vi "lock-in data transfer 0.3 copy.vi"(4 "points in buffer":i32=256, 5 "string":string="\n", 6 "number of points":dbl=617.0) -> (1 "Average\n[Y.0]":dbl, 2 "Average\n[X, R]":dbl, 3 "Array x":dbl[](array[numeric])=[0.0002212534, 0.0002746601, 0.0002899189, 0.0002365122, 0.0002441425, 0.0002555866, 0.0002059946, 0.0002021799, 0.0002594013, 0.0002594013, 0.0002288828, 0.0002708454, 0.0002937336, 0.0002479572, 0.0002365122, 0.000263216, 0.0002174387, 0.0001792917, 0.0002212534, 0.0002594013, 0.0002326975, 0.0002441425, 0.0002899189, 0.0002708454, 0.0002365122, 0.0002441425, 0.0002746601, 0.0002365122, 0.0002250681, 0.0002746601, 0.0002746601, 0.0002403269, 0.0002746601, 0.0002861042, 0.0002365122, 0.000213624, 0.0002555866, 0.0002250681, 0.0002174387, 0.0002937336, 0.000263216, 0.0002212534, 0.0002670307, 0.0003166217, 0.0002288828, 0.0002212534, 0.0002746601, 0.0003242511, 0.0002174387, 0.0002288828, 0.0003318805, 0.0002899189, 0.0002059946, 0.0002822895, 0.0002899189, 0.000213624, 0.0002098093, 0.000263216, 0.0002365122, 0.0002212534, 0.0002899189, 0.0002937336, 0.0002479572, 0.0002403269, 0.0002937336, 0.0002670307, 0.0002059946, 0.0002365122, 0.0002861042, 0.0002517719, 0.0002403269, 0.0002975482, 0.0002784748, 0.0002326975, 0.000263216, 0.0002861042, 0.000213624, 0.0001869211, 0.0002365122, 0.0002288828, 0.0002021799, 0.000263216, 0.0002861042, 0.0002365122, 0.0002403269, 0.0002937336, 0.0002708454, 0.0002326975, 0.000263216, 0.0002594013, 0.0002250681, 0.0002365122, 0.0002975482, 0.0002555866, 0.0002250681, 0.0002517719, 0.0002403269, 0.0002021799, 0.0002174387, 0.0002403269, 0.0002288828, 0.000213624, 0.000263216, 0.0002899189, 0.0002479572, 0.0002479572, 0.000263216, 0.0002365122, 0.0001831064, 0.0002441425, 0.0002746601, 0.0002365122, 0.0002441425, 0.0002975482, 0.0002670307, 0.0002212534, 0.0002403269, 0.0002517719, 0.0002098093, 0.0001945505, 0.0002288828, 0.0002326975, 0.0002326975, 0.0002784748, 0.0002861042, 0.0002403269, 0.0002479572, 0.0002822895, 0.0002517719, 0.0002098093, 0.0002670307, 0.0002784748, 0.0002365122, 0.0002517719, 0.0002975482, 0.0002746601, 0.0002365122, 0.0002555866, 0.0001983652, 0.000213624, 0.0002326975, 0.0002594013, 0.0002899189, 0.0002403269, 0.0002517719, 0.0003051776, 0.0002441425, 0.000263216, 0.0002746601, 0.0002555866, 0.0002326975, 0.0002365122, 0.000263216, 0.0002670307, 0.0002670307, 0.0002517719, 0.0002670307, 0.0002365122, 0.0002479572, 0.0002670307, 0.0002365122, 0.0002098093, 0.0002670307, 0.0002937336, 0.0002365122, 0.0002670307, 0.0002937336, 0.0002059946, 0.0002365122, 0.000312807, 0.0002403269, 0.0002174387, 0.0002784748, 0.0002899189, 0.0002250681, 0.0002746601, 0.000312807, 0.0002708454, 0.0002098093, 0.0002822895, 0.0003013629, 0.0002098093, 0.0002288828, 0.0003051776, 0.000263216, 0.0002288828, 0.0002822895, 0.0002822895, 0.0002365122, 0.0002365122, 0.0002937336, 0.0002594013, 0.0002288828, 0.0002899189, 0.0002937336, 0.0002365122, 0.0002479572, 0.0002861042, 0.0002365122, 0.000213624, 0.000263216, 0.0002670307, 0.0002288828, 0.000263216, 0.0002937336, 0.0002594013, 0.0002441425, 0.0002822895, 0.000263216, 0.0002021799, 0.000213624, 0.0002517719, 0.0002365122, 0.0002212534, 0.0002708454, 0.0002937336, 0.0002441425, 0.0002555866, 0.0002861042, 0.0002365122, 0.0002250681, 0.0002441425, 0.0002555866, 0.000213624, 0.0002517719, 0.0002861042, 0.0002555866, 0.0002365122, 0.0002670307, 0.0002479572, 0.0002059946, 0.0002479572, 0.0002746601, 0.0002326975, 0.0002250681, 0.0002899189, 0.0002746601, 0.0002441425, 0.000263216, 0.0002784748, 0.000213624, 0.0002098093, 0.0002555866, 0.000263216, 0.0002288828, 0.000263216, 0.0002784748, 0.0002441425, 0.0002288828, 0.0002708454, 0.000263216, 0.0001831064, 0.000213624, 0.0002441425, 0.0002594013, 0.0002555866, 0.0002670307, 0.0002708454, 0.0001869211, 0.000263216, 0.0003166217, 0.0002288828, 0.000213624, 0.0002975482, 0.0002822895, 0.0002212534, 0.0002861042, 0.0003089923, 0.0002326975, 0.0001945505, 0.0002250681, 0.0002975482, 0.0002212534, 0.0002250681, 0.0002708454, 0.0002784748, 0.0002365122, 0.000263216, 0.000312807, 0.0002365122, 0.0002365122, 0.0002899189, 0.0002670307, 0.000213624, 0.0002937336, 0.0002899189, 0.000213624, 0.0002441425, 0.0002899189, 0.0002403269, 0.0002250681, 0.0003013629, 0.0002899189, 0.0002250681, 0.0002365122, 0.0002899189, 0.000263216, 0.0002441425, 0.0002746601, 0.0002746601, 0.0002403269, 0.0002517719, 0.0002861042, 0.0002746601, 0.0002174387, 0.0003051776, 0.000312807, 0.0002365122, 0.0002403269, 0.0003013629, 0.0002670307, 0.0001983652, 0.0002861042, 0.0002784748, 0.0001945505, 0.0002517719, 0.0003089923, 0.0002326975, 0.0002288828, 0.000312807, 0.0003013629, 0.0002098093, 0.000263216, 0.0002784748, 0.0002517719, 0.000213624, 0.0002479572, 0.0003013629, 0.0002479572, 0.000213624, 0.0002746601, 0.0002365122, 0.0002059946, 0.0002365122, 0.0002670307, 0.0002288828, 0.0002174387, 0.0002822895, 0.000263216, 0.0002365122, 0.0002899189, 0.0002555866, 0.0002021799, 0.0002288828, 0.0002670307, 0.0002212534, 0.0002250681, 0.0002822895, 0.0002746601, 0.0002098093, 0.000263216, 0.0002746601, 0.0002098093, 0.0001907358, 0.0002441425, 0.0002479572, 0.0001945505, 0.0002555866, 0.0003051776, 0.0002365122, 0.0002365122, 0.0002784748, 0.0002479572, 0.0002098093, 0.0002403269, 0.0002746601, 0.0002326975, 0.0002441425, 0.0003013629, 0.0002784748, 0.0002212534, 0.0002517719, 0.0002594013, 0.0002059946, 0.0001983652, 0.0002555866, 0.0002594013, 0.0002365122, 0.000263216, 0.0002937336, 0.000263216, 0.0002479572, 0.0002784748, 0.0002555866, 0.0002288828, 0.0002479572, 0.0002708454, 0.0002365122, 0.0002555866, 0.0002746601, 0.0002555866, 0.0002288828, 0.0002517719, 0.0002670307, 0.0002212534, 0.0002326975, 0.0002594013, 0.0002555866, 0.0002326975, 0.0002746601, 0.0002899189, 0.0002517719, 0.0002288828, 0.0002670307, 0.0002403269, 0.0002174387, 0.000263216, 0.0002899189, 0.0002403269, 0.0002555866, 0.0002899189, 0.0002670307, 0.0002250681, 0.0002822895, 0.0002021799, 0.0001640329, 0.0002899189, 0.0002708454, 0.0001831064, 0.0002670307, 0.0003089923, 0.0002555866, 0.0002288828, 0.0002784748, 0.0002670307, 0.0002365122, 0.0002326975, 0.0002517719, 0.0002479572, 0.0002594013, 0.0002441425, 0.0002708454, 0.000263216, 0.0001831064, 0.0002517719, 0.0003242511, 0.0002059946, 0.0002479572, 0.0002746601, 0.0002365122, 0.0002555866, 0.0002937336, 0.0002708454, 0.0002250681, 0.0002555866, 0.0002746601, 0.0002098093, 0.0002365122, 0.0002937336, 0.0002594013, 0.000213624, 0.0002670307, 0.0002784748, 0.0002059946, 0.0002098093, 0.0003013629, 0.0002326975, 0.0001487741, 0.0002746601, 0.0002937336, 0.0002174387, 0.0002441425, 0.0002708454, 0.0002365122, 0.0002212534, 0.0002021799, 0.0001831064, 0.0002746601, 0.0002746601, 0.0002098093, 0.0002708454, 0.0002822895, 0.0002403269, 0.0002365122, 0.0002250681, 0.0001602182, 0.0002517719, 0.0002098093, 0.0002174387, 0.0002098093, 0.0002670307, 0.0002937336, 0.0002174387, 0.0002746601, 0.0002975482, 0.0002326975, 0.0002212534, 0.0002594013, 0.0002479572, 0.0002174387, 0.0002670307, 0.0002861042, 0.0002326975, 0.0002441425, 0.0002784748, 0.0002441425, 0.0002212534, 0.0002555866, 0.0002594013, 0.0002365122, 0.0002479572, 0.0002899189, 0.0002555866, 0.0002365122, 0.0002670307, 0.0002708454, 0.0002326975, 0.0002479572, 0.0002899189, 0.0002517719, 0.0002326975, 0.0002822895, 0.0002899189, 0.0002365122, 0.0002517719, 0.0002822895, 0.0002594013, 0.000213624, 0.0002746601, 0.0002861042, 0.0002365122, 0.0002594013, 0.0002937336, 0.0002555866, 0.0002250681, 0.0002822895, 0.0002861042, 0.0002250681, 0.0002517719, 0.0002975482, 0.0002555866, 0.0002365122, 0.0002899189, 0.000263216, 0.0002250681, 0.0002517719, 0.0002365122, 0.0002174387, 0.000263216, 0.0002746601, 0.0002708454, 0.0002326975, 0.0002479572, 0.0002822895, 0.0002708454, 0.0002250681, 0.0002365122, 0.0002594013, 0.0002365122, 0.0002479572, 0.0002517719, 0.0002784748, 0.000263216, 0.0002212534, 0.0002365122, 0.0002326975, 0.000263216, 0.0002594013, 0.0001869211, 0.0001831064, 0.0002899189, 0.0002899189, 0.000213624, 0.0002670307, 0.0002937336, 0.0001716623, 0.0001716623, 0.0003051776, 0.0002708454, 0.0001831064, 0.0002517719, 0.0002937336, 0.0002365122, 0.0002365122, 0.000263216, 0.0001792917, 0.0002098093, 0.0002212534, 0.000213624, 0.0002403269, 0.0001907358, 0.0002517719, 0.0002822895, 0.0002479572, 0.0002365122, 0.000263216, 0.0002288828, 0.0002365122, 0.000263216, 0.0002517719, 0.0002403269, 0.0002517719, 0.0002708454, 0.0002555866, 0.0001907358, 0.0002861042, 0.0002365122, 0.0001029973, 0.0002555866, 0.0003471393, 0.0001869211, 0.0002212534, 0.0003318805, 0.0002822895, 0.0002059946, 0.0002937336, 0.0003051776, 0.0001945505, 0.0002059946, 0.0003166217, 0.0002822895, 0.0001907358, 0.0002899189, 0.0002899189, 0.0001831064, 0.0002365122, 0.0002899189] format="%#_9e")   [LabVIEW 2010]
uses:
  Instance           1 38Saved   lock-in data transfer 0.3 copy .vi
  Instance           3 38Saved   lock-in data transfer 0.3 copy .vi
  Instance           2 38Saved   lock-in data transfer 0.3 copy .vi
  Instance           7 38Saved   lock-in data transfer 0.3 copy .vi
  Instance           6 38Saved   lock-in data transfer 0.3 copy .vi
  Instance          10 38Saved   lock-in data transfer 0.3 copy .vi
  Instance           5 38Saved   lock-in data transfer 0.3 copy .vi
  Instance           4 38Saved   lock-in data transfer 0.3 copy .vi
panel:
  out "Array y":dbl[](array[numeric])
  out "read \nbuffer 2":string="2.899189e-004,2.365122e-004,2.517719e-004,2.822895e-004,2.594013e-004,2.136240e-004,2.746601e-004,2.861042e-004,2.365122e-004,2.594013e-004,2.937336e-004,2.555866e-004,2.250681e-004,2.822895e-004,2.861042e-004,2.250681e-004,2.517719e-004,2.975482e-004,2.555866e-004,2.365122e-004,2.899189e-004,2.632160e-004,2.250681e-004,2.517719e-004,2.365122e-004,2.174387e-004,2.632160e-004,2.746601e-004,2.708454e-004,2.326975e-004,2.479572e-004,2.822895e-004,2.708454e-004,2.250681e-004,2.365122e-004,2.594013e-004,2.365122e-004,2.479572e-004,2.517719e-004,2.784748e-004,2.632160e-004,2.212534e-004,2.365122e-004,2.326975e-004,2.632160e-004,2.594013e-004,1.869211e-004,1.831064e-004,2.899189e-004,2.899189e-004,2.136240e-004,2.670307e-004,2.937336e-004,1.716623e-004,1.716623e-004,3.051776e-004,2.708454e-004,1.831064e-004,2.517719e-004,2.937336e-004,2.365122e-004,2.365122e-004,2.632160e-004,1.792917e-004,2.098093e-004,2.212534e-004,2.136240e-004,2.403269e-004,1.907358e-004,2.517719e-004,2.822895e-004,2.479572e-004,2.365122e-004,2.632160e-004,2.288828e-004,2.365122e-004,2.632160e-004,2.517719e-004,2.403269e-004,2.517719e-004,2.708454e-004,2.555866e-004,1.907358e-004,2.861042e-004,2.365122e-004,1.029973e-004,2.555866e-004,3.471393e-004,1.869211e-004,2.212534e-004,3.318805e-004,2.822895e-004,2.059946e-004,2.937336e-004,3.051776e-004,1.945505e-004,2.059946e-004,3.166217e-004,2.822895e-004,1.907358e-004,2.899189e-004,2.899189e-004,1.831064e-004,2.365122e-004,2.899189e-004,\n"
  out "read\nbuffer":string="2.899189e-004,2.365122e-004,2.517719e-004,2.822895e-004,2.594013e-004,2.136240e-004,2.746601e-004,2.861042e-004,2.365122e-004,2.594013e-004,2.937336e-004,2.555866e-004,2.250681e-004,2.822895e-004,2.861042e-004,2.250681e-004,2.517719e-004,2.975482e-004,2.555866e-004,2.365122e-004,2.899189e-004,2.632160e-004,2.250681e-004,2.517719e-004,2.365122e-004,2.174387e-004,2.632160e-004,2.746601e-004,2.708454e-004,2.326975e-004,2.479572e-004,2.822895e-004,2.708454e-004,2.250681e-004,2.365122e-004,2.594013e-004,2.365122e-004,2.479572e-004,2.517719e-004,2.784748e-004,2.632160e-004,2.212534e-004,2.365122e-004,2.326975e-004,2.632160e-004,2.594013e-004,1.869211e-004,1.831064e-004,2.899189e-004,2.899189e-004,2.136240e-004,2.670307e-004,2.937336e-004,1.716623e-004,1.716623e-004,3.051776e-004,2.708454e-004,1.831064e-004,2.517719e-004,2.937336e-004,2.365122e-004,2.365122e-004,2.632160e-004,1.792917e-004,2.098093e-004,2.212534e-004,2.136240e-004,2.403269e-004,1.907358e-004,2.517719e-004,2.822895e-004,2.479572e-004,2.365122e-004,2.632160e-004,2.288828e-004,2.365122e-004,2.632160e-004,2.517719e-004,2.403269e-004,2.517719e-004,2.708454e-004,2.555866e-004,1.907358e-004,2.861042e-004,2.365122e-004,1.029973e-004,2.555866e-004,3.471393e-004,1.869211e-004,2.212534e-004,3.318805e-004,2.822895e-004,2.059946e-004,2.937336e-004,3.051776e-004,1.945505e-004,2.059946e-004,3.166217e-004,2.822895e-004,1.907358e-004,2.899189e-004,2.899189e-004,1.831064e-004,2.365122e-004,2.899189e-004,\n"
  out "size":i32=617
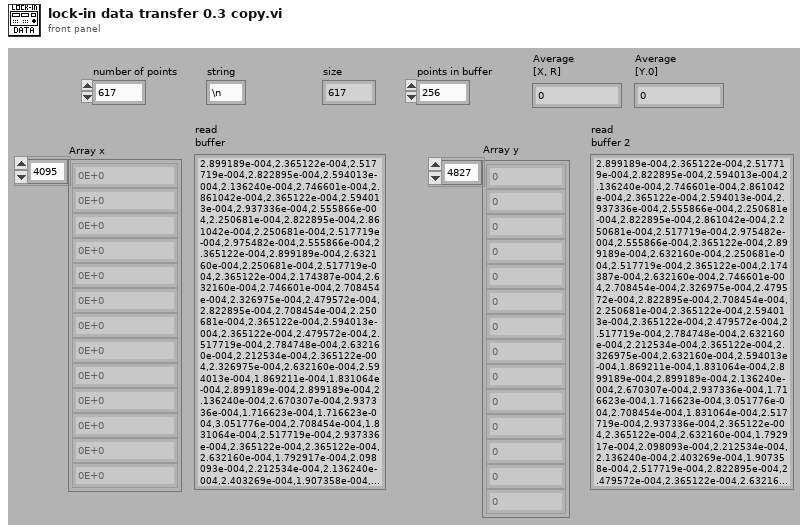
[diagram p1: front panel]
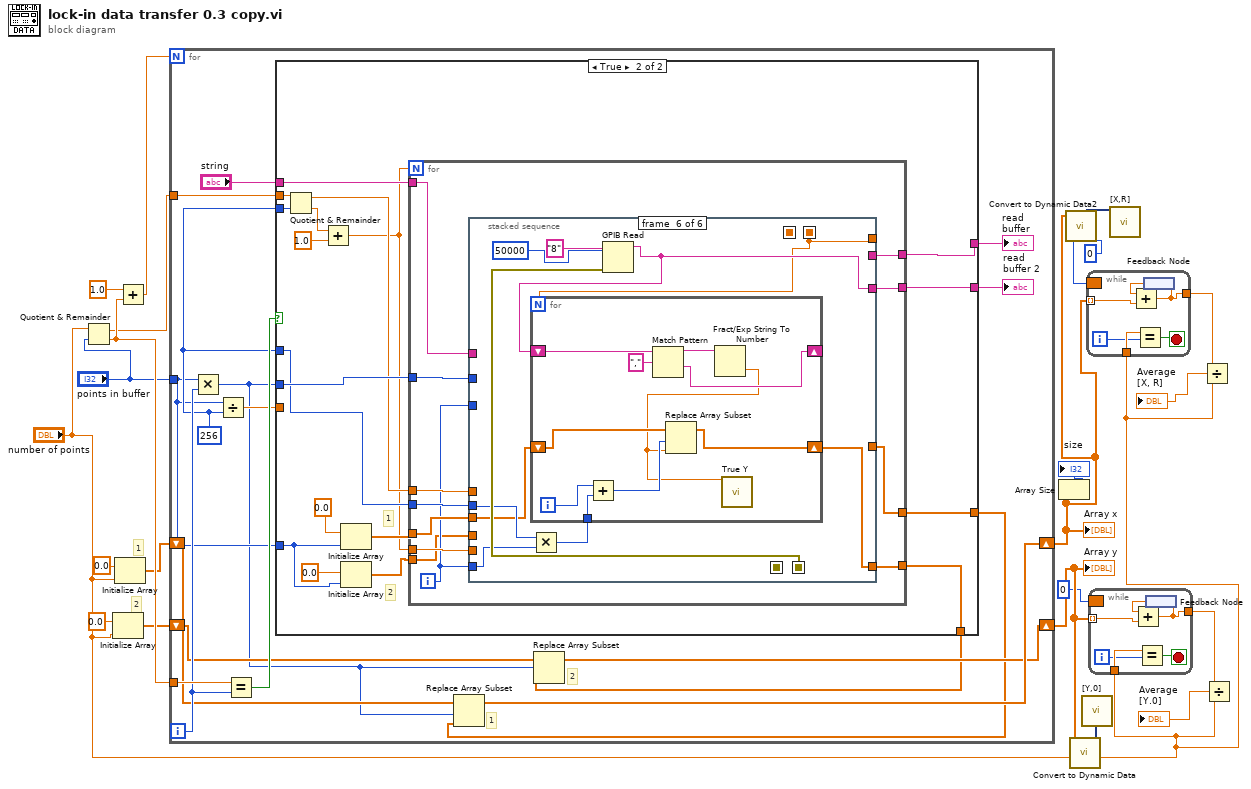
[diagram p0: block diagram]
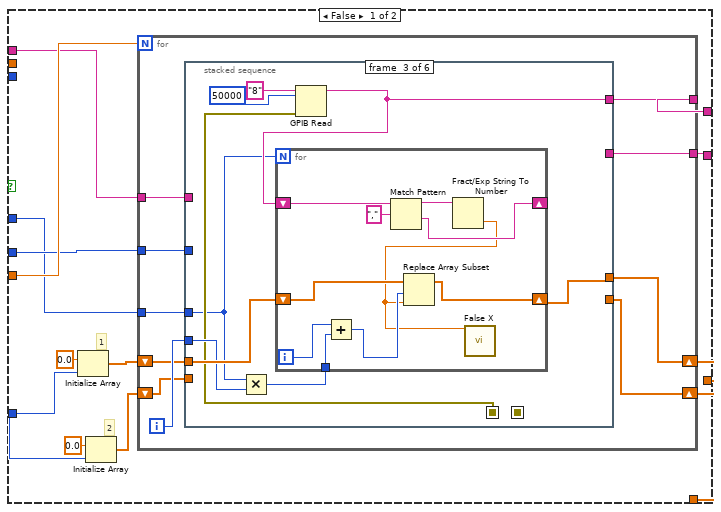
[diagram p2: hidden frame]
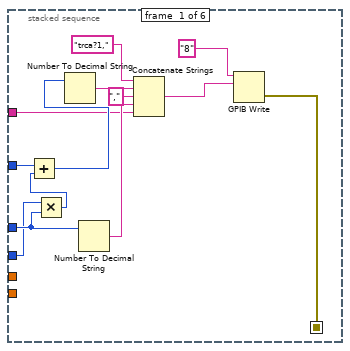
[diagram p3: hidden frame]
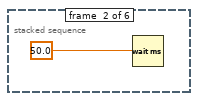
[diagram p4: hidden frame]
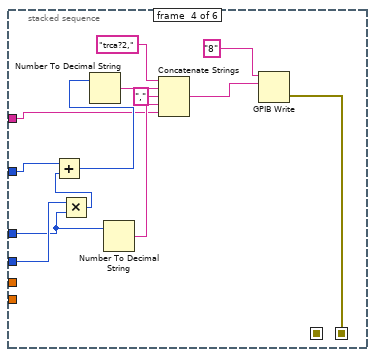
[diagram p5: hidden frame]
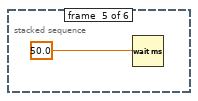
[diagram p6: hidden frame]
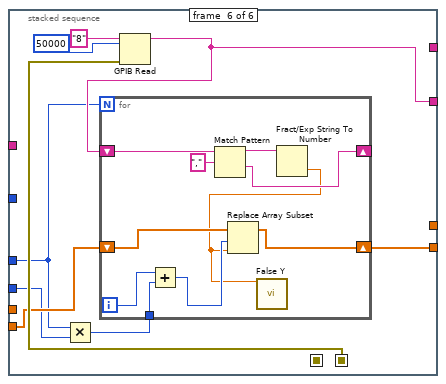
[diagram p7: hidden frame]
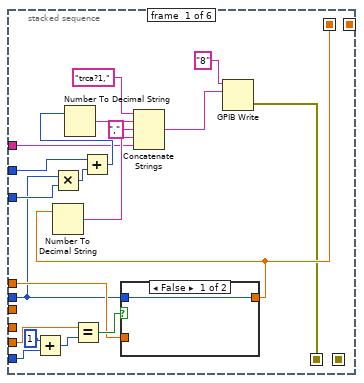
[diagram p8: hidden frame]
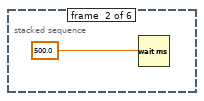
[diagram p10: hidden frame]
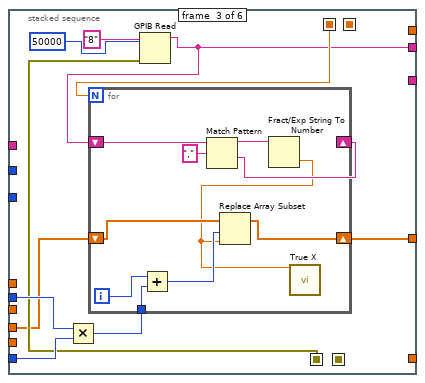
[diagram p11: hidden frame]
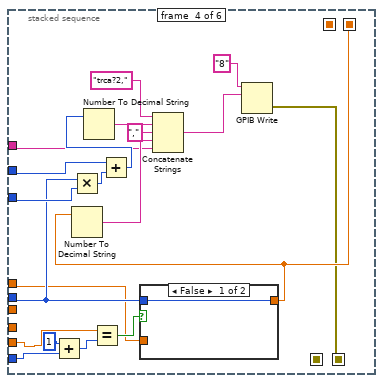
[diagram p12: hidden frame]
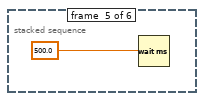
[diagram p14: hidden frame]
diagram:
  # "2"
  # "1"
  n1 = Quotient & Remainder(x="number of points", y="points in buffer") -> (x-y*floor(x/y)=w14:dbl, floor(x/y)=w19:dbl)
  n2 = Initialize Array(0.0 ("element"), "number of points") -> (w12:dbl[])
  n3 = Initialize Array(0.0 ("element"), "number of points") -> (w16:dbl[])
  n4 = Add(x=1.0, y=w19) -> (x+y=w20:dbl)
  n5 = for {
    N: w20 -> [_]
    tunnel: "points in buffer" -> [w30]
    tunnel: w19 -> [w38]
    shift-right: [w35] -> w7
    shift-left: w16 -> [w36]
    tunnel: w14 -> [w33]
    shift-right: [w26] -> w10
    shift-left: w12 -> [w27]
    i -> [w37]
    w32 = 256
    # "2"
    # "1"
    n6 = Multiply(x=w30, y=w37) -> (x*y=w25:i32)
    n7 = Divide(x=w30, y=w32) -> (x/y=w31:dbl)
    n8 = Equal?(x=w38, y=w37) -> (x = y?=w34:bool)
    n9 = case shown="True" w34 {
      tunnel: w32 -> [w48 w138]
      tunnel: w33 -> [_ w145]
      tunnel: w32 -> [_ w144]
      tunnel: w31 -> [w51 _]
      tunnel: w25 -> [w50 w143]
      tunnel: [w47 w136] -> w22
      tunnel: w30 -> [w41 w132]
      tunnel: "string" -> [w46 w135]
      tunnel: [w45 w134] -> w28
      tunnel: [w43 w128] -> w24
      tunnel: [w39 w130] -> w23
      frame False {
        # "2"
        # "1"
        n10 = Initialize Array(0.0 ("element"), w41) -> (w44:dbl[])
        n11 = Initialize Array(0.0 ("element"), w41) -> (w40:dbl[])
        n12 = for {
          N: w51 -> [_]
          tunnel: w48 -> [w60]
          tunnel: w50 -> [w59]
          tunnel: w46 -> [w58]
          tunnel: [w57] -> w45
          shift-right: [w53] -> w47
          shift-left: w44 -> [w56]
          tunnel: [w55] -> w43
          shift-right: [w52] -> w39
          shift-left: w40 -> [w54]
          i -> [w61]
          n13 = stacked-sequence {
            seq-local: [w62 _ _ _ _ _] -> [_ _ w79 _ _ _]
            seq-local: [_ _ _ w95 _ _] -> [_ _ _ _ _ w113]
            tunnel: w61 -> [w69 _ w82 w97 _ w110]
            tunnel: w56 -> [_ _ w84 _ _ _]
            tunnel: [_ _ w83 _ _ _] -> w53
            tunnel: w60 -> [w70 _ w76 w96 _ w111]
            tunnel: w59 -> [w68 _ _ w98 _ _]
            tunnel: w58 -> [w65 _ _ w99 _ _]
            tunnel: [_ _ w78 _ _ _] -> w57
            tunnel: [_ _ _ _ _ w114] -> w55
            tunnel: w54 -> [_ _ _ _ _ w112]
            tunnel: [_ _ _ _ _ w109] -> w52
            frame #0 {
              n14 = Multiply(x=w69, y=w70) -> (x*y=w67:i32)
              n15 = Add(x=w68, y=w67) -> (x+y=w66:i32)
              n16 = Number To Decimal String(number=w66) -> (decimal integer string=w73:string)  [unwired: 1 out]
              n17 = Number To Decimal String(number=w70) -> (decimal integer string=w71:string)  [unwired: 1 out]
              n18 = Concatenate Strings("trca?1,", w73, "," ("string"), w71, w65) -> (w63:string)
              n19 = GPIB Write(0:"8", 1:w63) -> (6:w62:errorcluster)  [unwired: 1 in, 3 out]
            }
            frame #1 {
              n20 = Wait (ms)(milliseconds to wait=50.0 ("x")) -> ()  [unwired: 1 out]
            }
            frame #2 {
              n21 = Multiply(x=w76, y=w82) -> (x*y=w81:i32)
              n22 = GPIB Read(0:"8", 1:50000, 3:w79) -> (5:w78:string)  [unwired: 4 out]
              n23 = for {
                N: w76 -> [_]
                shift-right: [w90] -> _
                shift-left: w78 -> [w92]
                shift-right: [w89] -> w83
                shift-left: w84 -> [w91]
                tunnel: w81 -> [w88]
                i -> [w87]
                n24 = Add(x=w87, y=w88) -> (x+y=w86:i32)
                n25 = Match Pattern(string=w92, regular expression=",") -> (before substring=w94:string, after substring=w90:string)  [unwired: 3 out]
                n26 = Fract/Exp String To Number(string=w94) -> (number=w85:dbl)  [unwired: 4 out]
                n27 = Replace Array Subset(array=w91, new element=w85, index=w86) -> (w89:dbl[])
                n28 = call "False X"("Signals"=w85) -> ()  [unwired: 6 in, 13 out]
              }
            }
            frame #3 {
              n29 = Multiply(x=w97, y=w96) -> (x*y=w104:i32)
              n30 = Add(x=w98, y=w104) -> (x+y=w105:i32)
              n31 = Number To Decimal String(number=w105) -> (decimal integer string=w101:string)  [unwired: 1 out]
              n32 = Number To Decimal String(number=w96) -> (decimal integer string=w103:string)  [unwired: 1 out]
              n33 = Concatenate Strings("trca?2,", w101, "," ("string"), w103, w99) -> (w107:string)
              n34 = GPIB Write(0:"8", 1:w107) -> (6:w95:errorcluster)  [unwired: 1 in, 3 out]
            }
            frame #4 {
              n35 = Wait (ms)(milliseconds to wait=50.0 ("x")) -> ()  [unwired: 1 out]
            }
            frame #5 {
              n36 = Multiply(x=w111, y=w110) -> (x*y=w117:i32)
              n37 = GPIB Read(0:"8", 1:50000, 3:w113) -> (5:w114:string)  [unwired: 4 out]
              n38 = for {
                N: w111 -> [_]
                shift-right: [w123] -> _
                shift-left: w114 -> [w125]
                shift-right: [w122] -> w109
                shift-left: w112 -> [w124]
                tunnel: w117 -> [w121]
                i -> [w120]
                n39 = Add(x=w120, y=w121) -> (x+y=w119:i32)
                n40 = Match Pattern(string=w125, regular expression=",") -> (before substring=w127:string, after substring=w123:string)  [unwired: 3 out]
                n41 = Fract/Exp String To Number(string=w127) -> (number=w118:dbl)  [unwired: 4 out]
                n42 = Replace Array Subset(array=w124, new element=w118, index=w119) -> (w122:dbl[])
                n43 = call "False Y"("Signals"=w118) -> ()  [unwired: 6 in, 13 out]
              }
            }
          }
        }
      }
      frame True {
        # "2"
        # "1"
        n44 = Quotient & Remainder(x=w145, y=w144) -> (x-y*floor(x/y)=w141:dbl, floor(x/y)=w140:dbl)
        n45 = Add(x=w140, y=1.0) -> (x+y=w129:dbl)
        n46 = Initialize Array(0.0 ("element"), w132) -> (w137:dbl[])
        n47 = Initialize Array(0.0 ("element"), w132) -> (w131:dbl[])
        n48 = for {
          N: w129 -> [_]
          tunnel: w143 -> [w157]
          tunnel: w129 -> [w155]
          tunnel: w138 -> [w154]
          tunnel: w141 -> [w153]
          tunnel: w137 -> [w156]
          tunnel: [w147] -> w136
          tunnel: w135 -> [w151]
          tunnel: [w150] -> w134
          tunnel: [w149] -> w128
          tunnel: w131 -> [w148]
          tunnel: [w146] -> w130
          i -> [w152]
          n49 = stacked-sequence {
            seq-local: [w158 _ _ _ _ _] -> [_ _ w186 _ _ _]
            seq-local: [w162 _ _ _ _ _] -> [_ _ w184 _ _ _]
            seq-local: [_ _ _ w203 _ _] -> [_ _ _ _ _ w225]
            seq-local: [_ _ _ w202 _ _] -> [_ _ _ _ _ w230]
            tunnel: w157 -> [w164 _ _ w208 _ _]
            tunnel: w156 -> [_ _ _ _ _ w224]
            tunnel: [_ _ w181 _ _ _] -> w147
            tunnel: w152 -> [w173 _ w189 w201 _ w226]
            tunnel: w155 -> [w170 _ _ w206 _ _]
            tunnel: w154 -> [w166 _ w190 w205 _ w229]
            tunnel: w153 -> [w168 _ _ w204 _ _]
            tunnel: w152 -> [w167 _ _ w207 _ _]
            tunnel: w151 -> [w161 _ _ w209 _ _]
            tunnel: [_ _ w182 _ _ _] -> w150
            tunnel: [_ _ _ _ _ w228] -> w149
            tunnel: w148 -> [_ _ w183 _ _ _]
            tunnel: [_ _ _ _ _ w227] -> w146
            tunnel: [_ _ _ _ _ w225] -> _
            frame #0 {
              n50 = Add(x=1, y=w173) -> (x+y=w171:i32)
              n51 = Multiply(x=w166, y=w167) -> (x*y=w165:i32)
              n52 = Equal?(x=w170, y=w171) -> (x = y?=w169:bool)
              n53 = Add(x=w164, y=w165) -> (x+y=w163:i32)
              n54 = Number To Decimal String(number=w163) -> (decimal integer string=w176:string)  [unwired: 1 out]
              n55 = case shown="False" w169 {
                tunnel: [w178 w179] -> w162
                tunnel: w166 -> [w178 _]
                tunnel: w168 -> [_ w179]
                frame False {
                }
                frame True {
                }
              }
              n56 = Number To Decimal String(number=w162) -> (decimal integer string=w174:string)  [unwired: 1 out]
              n57 = Concatenate Strings("trca?1,", w176, "," ("string"), w174, w161) -> (w159:string)
              n58 = GPIB Write(0:"8", 1:w159) -> (6:w158:errorcluster)  [unwired: 1 in, 3 out]
            }
            frame #1 {
              n59 = Wait (ms)(milliseconds to wait=500.0 ("x")) -> ()  [unwired: 1 out]
            }
            frame #2 {
              n60 = Multiply(x=w190, y=w189) -> (x*y=w188:i32)
              n61 = GPIB Read(0:"8", 1:50000, 3:w186) -> (5:w182:string)  [unwired: 4 out]
              n62 = for {
                N: w184 -> [_]
                shift-right: [w196] -> _
                shift-left: w182 -> [w198]
                shift-right: [w195] -> w181
                shift-left: w183 -> [w197]
                tunnel: w188 -> [w194]
                i -> [w193]
                n63 = Add(x=w193, y=w194) -> (x+y=w192:i32)
                n64 = Match Pattern(string=w198, regular expression=",") -> (before substring=w200:string, after substring=w196:string)  [unwired: 3 out]
                n65 = Fract/Exp String To Number(string=w200) -> (number=w191:dbl)  [unwired: 4 out]
                n66 = Replace Array Subset(array=w197, new element=w191, index=w192) -> (w195:dbl[])
                n67 = call "True X"("Signals"=w191) -> ()  [unwired: 6 in, 13 out]
              }
            }
            frame #3 {
              n68 = Add(x=1, y=w201) -> (x+y=w215:i32)
              n69 = Multiply(x=w205, y=w207) -> (x*y=w213:i32)
              n70 = Equal?(x=w206, y=w215) -> (x = y?=w214:bool)
              n71 = Add(x=w208, y=w213) -> (x+y=w212:i32)
              n72 = Number To Decimal String(number=w212) -> (decimal integer string=w219:string)  [unwired: 1 out]
              n73 = case shown="False" w214 {
                tunnel: [w221 w222] -> w203
                tunnel: w205 -> [w221 _]
                tunnel: w204 -> [_ w222]
                frame False {
                }
                frame True {
                }
              }
              n74 = Number To Decimal String(number=w203) -> (decimal integer string=w217:string)  [unwired: 1 out]
              n75 = Concatenate Strings("trca?2,", w219, "," ("string"), w217, w209) -> (w210:string)
              n76 = GPIB Write(0:"8", 1:w210) -> (6:w202:errorcluster)  [unwired: 1 in, 3 out]
            }
            frame #4 {
              n77 = Wait (ms)(milliseconds to wait=500.0 ("x")) -> ()  [unwired: 1 out]
            }
            frame #5 {
              n78 = Multiply(x=w229, y=w226) -> (x*y=w231:i32)
              n79 = GPIB Read(0:"8", 1:50000, 3:w230) -> (5:w228:string)  [unwired: 4 out]
              n80 = for {
                N: w225 -> [_]
                shift-right: [w239] -> _
                shift-left: w228 -> [w241]
                shift-right: [w234] -> w227
                shift-left: w224 -> [w240]
                tunnel: w231 -> [w238]
                i -> [w237]
                n81 = Add(x=w237, y=w238) -> (x+y=w236:i32)
                n82 = Match Pattern(string=w241, regular expression=",") -> (before substring=w243:string, after substring=w239:string)  [unwired: 3 out]
                n83 = Fract/Exp String To Number(string=w243) -> (number=w235:dbl)  [unwired: 4 out]
                n84 = Replace Array Subset(array=w240, new element=w235, index=w236) -> (w234:dbl[])
                n85 = call "True Y"("Signals"=w235) -> ()  [unwired: 6 in, 13 out]
              }
            }
          }
        }
      }
    }
    "read\nbuffer" <- w28
    "read \nbuffer 2" <- w24
    n86 = Replace Array Subset(array=w36, new element=w22, index=w25) -> (w35:dbl[])
    n87 = Replace Array Subset(array=w27, new element=w23, index=w25) -> (w26:dbl[])
  }
  "Array x" <- w7
  "Array y" <- w10
  n88 = Array Size(array=w7) -> (size(s)=→"size":i32)
  n89 = call "Convert to Dynamic Data2"("Array"=w7) -> ("Dynamic Data Type"=w6:dynamicdata)  [unwired: 3 out]
  n90 = call "Convert to Dynamic Data"("Array"=w10) -> ("Dynamic Data Type"=w11:dynamicdata)  [unwired: 3 out]
  n91 = call "[Y,0]"("Signals"=w11) -> ()  [unwired: 6 in, 13 out]
  n92 = while {
    tunnel: "number of points" -> [w248]
    tunnel: w7 -> [w246] mode=indexing
    tunnel: [w244] -> w8
    border: 0 -> [_]
    i -> [w247]
    stop <- w249 stop-if-true
    n93 = Equal?(x=w248, y=w247) -> (x = y?=w249:bool)
    n94 = feedback #1() -> (w245:dbl)
    n95 = Add(x=w245, y=w246) -> (x+y=w244:dbl)
    n96 = feedback-in #1(w244) -> ()
  }
  n97 = while {
    tunnel: "number of points" -> [w254]
    tunnel: w10 -> [w252] mode=indexing
    tunnel: [w250] -> w9
    border: 0 -> [_]
    i -> [w253]
    stop <- w255 stop-if-true
    n98 = Equal?(x=w254, y=w253) -> (x = y?=w255:bool)
    n99 = feedback #2() -> (w251:dbl)
    n100 = Add(x=w251, y=w252) -> (x+y=w250:dbl)
    n101 = feedback-in #2(w250) -> ()
  }
  n102 = call "[X,R]"("Signals"=w6) -> ()  [unwired: 6 in, 13 out]
  n103 = Divide(x=w8, y="number of points") -> (x/y=→"Average\n[X, R]":dbl)
  n104 = Divide(x=w9, y="number of points") -> (x/y=→"Average\n[Y.0]":dbl)
